vi "FM Gen Pulse for FIB-SEM.vi"(7 "WatchDog Mode":u16(ring)=2 items=["Do Nothing", "Send Idle Only", "Watch FIB & SEM", "Watch FIB Only", "Watch SEM Only"], 8 "error in":errorcluster, 9 "watchdog counter":tag="Log/ctr0", 10 "watchdog FM":tag="/Log/PFI15", 11 "State Value":i16) -> (0 "error out":errorcluster, 2 "Burst length (mSec)":dbl, 3 "Actual Frequency":dbl)   [LabVIEW 2012]
doc: "This example demonstrates how to generate a finite number of digital pulses using a counter output.\n\nOn some hardware, this requires the use of a second counter to generate a gate signal. If necessary, DAQmx configures this second counter for you."
uses:
  <vilib>/DAQmx/create/channels.llb/DAQmx Create Channel (CO-Pulse Generation-Frequency).vi
  <vilib>/DAQmx/configure/timing.llb/DAQmx Timing (Implicit).vi
  <resource>/objmgr/daqmx.rc
panel:
  in  "Number of Pulses":i32=5
  in  "Duty Cycle":dbl=0.5 min=0.01 max=0.99 step=0.05 format="%.2f"
  # "State Values:\n-1: error state.  Solenoid is energized.\n0: Startup and program exit state\n1: idle, solenoid off.\n2: check FIB X scan in progress\n3: check FIB X end state\n4: check SEM Y scan in progress\n5: check SEM Y scan end state\n\nIf FIB-SEM has an error: cRIO State -1 \nenergizes solenoid and cRIO goes to \nstate 0.  User must issue cmd to exit \nstate 0 to state 1 before any other state \ncan be accessed again."
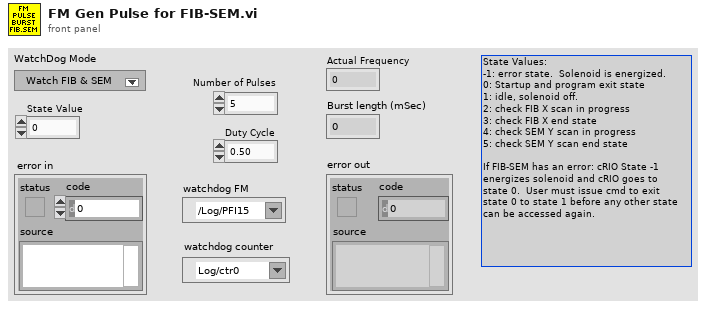
[diagram p1: front panel]
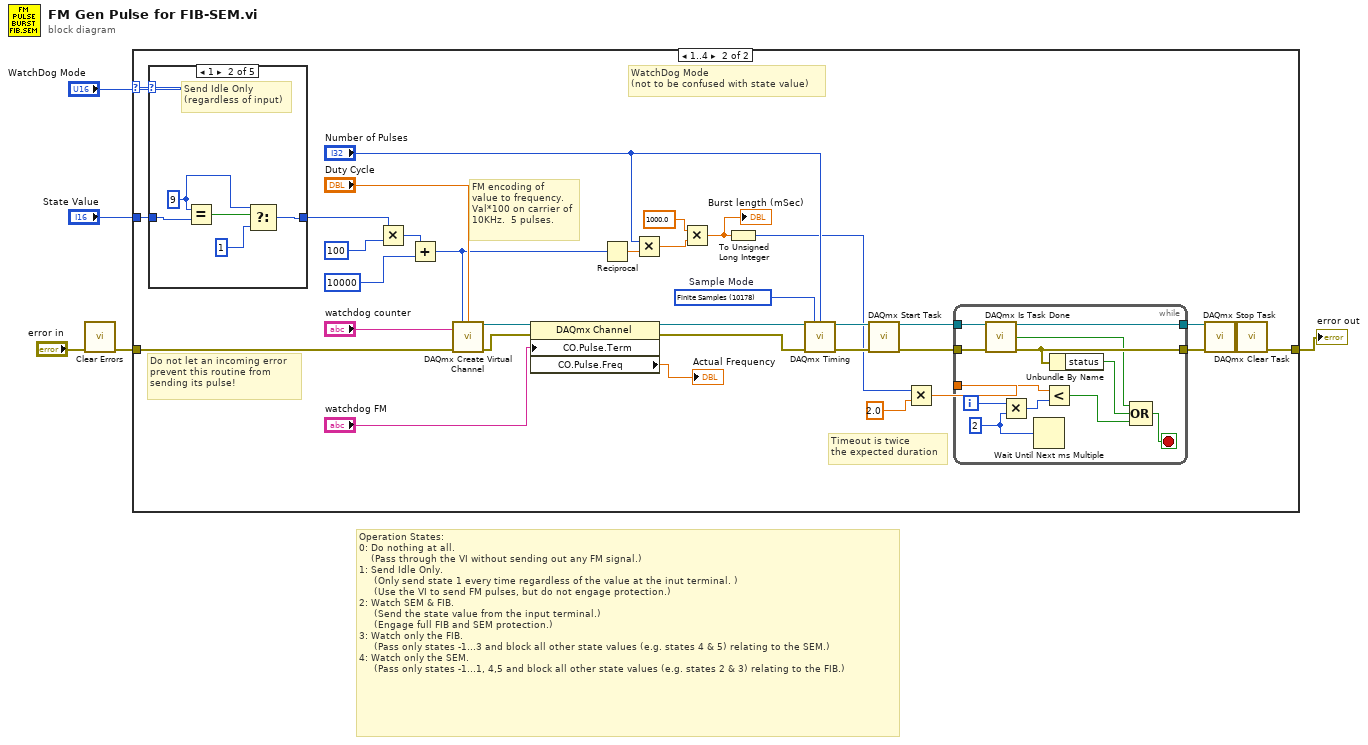
[diagram p0: block diagram]
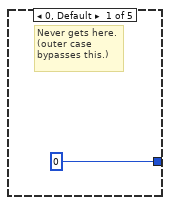
[diagram p3: hidden frame]
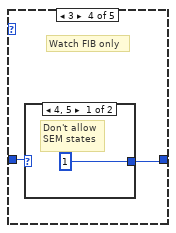
[diagram p5: hidden frame]
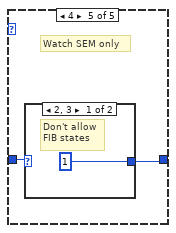
[diagram p7: hidden frame]
diagram:
  # "Operation States:\n0: Do nothing at all.  \n    (Pass through the VI without sending out any FM signal.)\n1: Send Idle Only. \n     (Only send state 1 every time regardless of the value at the inut terminal. )\n     (Use the VI to send FM pulses, but do not engage protection.)\n2: Watch SEM & FIB.\n     (Send the state value from the input terminal.)\n     (Engage full FIB and SEM protection.)\n3: Watch only the FIB. \n     (Pass only states -1...3 and block all other state values (e.g. states 4 & 5) relating to the SEM.)\n4: Watch only the SEM.\n     (Pass only states -1...1, 4,5 and block all other state values (e.g. states 2 & 3) relating to the FIB.)"
  n1 = call <vilib>:"Clear Errors.vi"("error in (no error)"="error in") -> ("error out"=w2:errorcluster)  [unwired: 6 in]
  n2 = case shown="1..4" "WatchDog Mode" {
    selector: "WatchDog Mode" -> [_ w11]
    tunnel: w2 -> [w6 w8]
    tunnel: "State Value" -> [_ w10]
    tunnel: [w6 w7] -> w1
    frame 0, Default {
      # "Do nothing at all.\nDon't even send FM pulses"
    }
    frame 1..4 {
      w40 = 10178 items=["Finite Samples"=10178, "Continuous Samples"=10123, "Hardware Timed Single Point"=12522]  # Sample Mode
      # "Do not let an incoming error\nprevent this routine from\nsending its pulse!"
      # "WatchDog Mode\n(not to be confused with state value)"
      # "FM encoding of\nvalue to frequency.\nVal*100 on carrier of\n10KHz.  5 pulses."
      # "Timeout is twice\nthe expected duration"
      n3 = case shown="1" w11 {
        tunnel: w10 -> [_ w46 w47 w49 w53]
        tunnel: [i16 0 ("State Value") w42 w47 w48 w52] -> w9
        frame 0, Default {
          # "Never gets here.\n(outer case\nbypasses this.)"
        }
        frame 1 {
          w44 = i16 9 ("x")
          # "Send Idle Only\n(regardless of input)"
          n4 = Equal?(x=w44, y=w46) -> (x = y?=w45:bool)
          n5 = Select(t=w44, s=w45, f=i16 1 ("State Value")) -> (s? t:f=w42:i16)
        }
        frame 2 {
          # "Normal Operation\nWatch FIB & SEM\n(send all FM states)"
        }
        frame 3 {
          # "Watch FIB only"
          n6 = case shown="4, 5" w49 {
            selector: w49 -> [_ w51]
            tunnel: [i16 1 ("State Value") w51] -> w48
            frame 4, 5 {
              # "Don't allow\nSEM states"
            }
            frame ..3, 6.., Default {
            }
          }
        }
        frame 4 {
          # "Watch SEM only"
          n7 = case shown="2, 3" w53 {
            selector: w53 -> [_ w55]
            tunnel: [i16 1 ("State Value") w55] -> w52
            frame 2, 3 {
              # "Don't allow\nFIB states"
            }
            frame ..1, 4.., Default {
            }
          }
        }
      }
      n8 = Multiply(x=w9, y=i16 100) -> (x*y=w14:i16)
      n9 = Add(x=w14, y=i16 10000) -> (x+y=w12:i16)
      n10 = call-poly <vilib>:"DAQmx Create Virtual Channel.vi"("frequency"=w12, "duty cycle"="Duty Cycle", "counter"="watchdog counter", "error in"=w8) -> ("task out"=w37:refnum<k21>, "error out"=w36:errorcluster)  [unwired: 10 in]
      n11 = property class="DAQmx Channel"(reference=w37, error in=w36, "CO.Pulse.Term"="watchdog FM") -> (reference out=w34:refnum<k21>, error out=w35:errorcluster, "CO.Pulse.Freq"=→"Actual Frequency":dbl)
      n12 = Reciprocal(x=w12) -> (1/x=w23:dbl)
      n13 = Multiply(x="Number of Pulses", y=w23) -> (x*y=w21:dbl)
      n14 = Multiply(x=1000.0, y=w21) -> (x*y=w16:dbl)
      "Burst length (mSec)" <- w16
      n15 = To Unsigned Long Integer(number=w16) -> (unsigned 32bit integer=w17:u32)
      n16 = call-poly <vilib>:"DAQmx Timing.vi"("task/channels in"=w34, "sample mode"=w40, "samples per channel"="Number of Pulses", "error in"=w35) -> ("task out"=w27:refnum<k21>, "error out"=w26:errorcluster)  [unwired: 10 in]
      n17 = call <vilib>:"DAQmx Start Task.vi"("task/channels in"=w27, "error in"=w26) -> ("task out"=w39:refnum<k21>, "error out"=w38:errorcluster)  [unwired: 12 in]
      n18 = Multiply(x=w17, y=2.0) -> (x*y=w18:dbl)
      n19 = while {
        tunnel: w39 -> [w67]
        tunnel: w38 -> [w66]
        tunnel: [w63] -> w28
        tunnel: [w64] -> w29
        tunnel: w18 -> [w56]
        i -> [w60]
        stop <- w65 stop-if-true
        w59 = u32 2 ("millisecond multiple")
        n20 = call <vilib>:"DAQmx Is Task Done.vi"("task/channels in"=w67, "error in"=w66) -> ("task out"=w64:refnum<k21>, "task done?"=w61:bool, "error out"=w63:errorcluster)  [unwired: 11 in]
        n21 = Multiply(x=w60, y=w59) -> (x*y=w58:u32)
        n22 = Wait Until Next ms Multiple(millisecond multiple=w59) -> ()  [unwired: 1 out]
        n23 = Less?(x=w56, y=w58) -> (x < y?=w57:bool)
        n24 = Unbundle By Name(w63) -> ("status"=w62:bool)
        n25 = Compound Arithmetic op=OR(w61, w62, w57) -> (w65:bool)
      }
      n26 = call <vilib>:"DAQmx Stop Task.vi"("task/channels in"=w29, "error in"=w28) -> ("task out"=w31:refnum<k21>, "error out"=w30:errorcluster)  [unwired: 12 in]
      n27 = call <vilib>:"DAQmx Clear Task.vi"("task in"=w31, "error in"=w30) -> ("error out"=w7:errorcluster)  [unwired: 13 in]
    }
  }
  "error out" <- w1
